vi "KE622x -- Set Current Level.vi"(0 "Resource In":refnum<visa-resource-name>, 1 "Check For SCPI Errors? (T)":bool=TRUE, 7 "Current Level (A) In":T1=0.1 min=-0.105 max=0.105 format="%.4p", 11 "error in (no error)":errorcluster, 12 "Read Back Set Value? (T)":bool=TRUE) -> (4 "Resource Out (dupl)":refnum<visa-resource-name>, 8 "Current Level (A) Out":T1=0.1 min=-0.105 max=0.105 format="%.4p", 15 "error out":errorcluster)   [LabVIEW 2019, in "Keithley 622x.lvlib"]
doc: "Sets the output current level when the source is operating in a DC mode (i.e. static mode)."
uses:
  Keithley 622x.lvlib
  Typedefs/KE622x -- Current Level.ctl
  Typedefs/KE622x -- Current Ranges.ctl
  Typedefs/KE622x -- Current Range.ctl
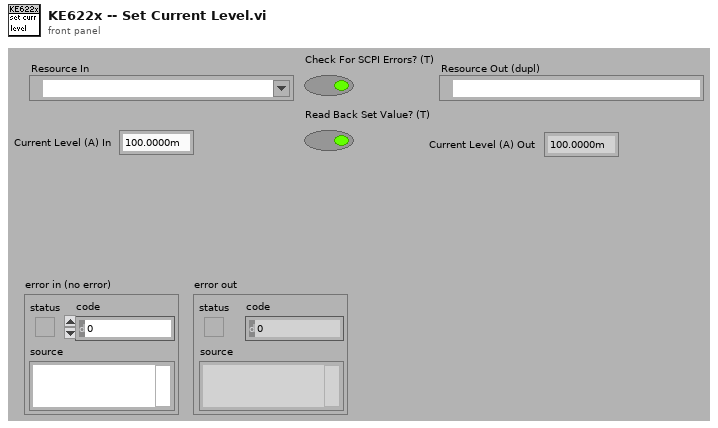
[diagram p1: front panel]
types:
  T1 = typedef "Keithley 622x.lvlib/KE622x -- Current Level.ctl" = dbl
  T2 = typedef "Keithley 622x.lvlib/KE622x -- Current Range.ctl" = cluster{"Auto Range?":bool, "Man / Selected\nRange":T3}
  T3 = typedef "Keithley 622x.lvlib/KE622x -- Current Ranges.ctl" = enum16{"2nA", "20nA", "200nA", "2uA", "20uA", "200uA", "2mA", "20mA", "100mA"}
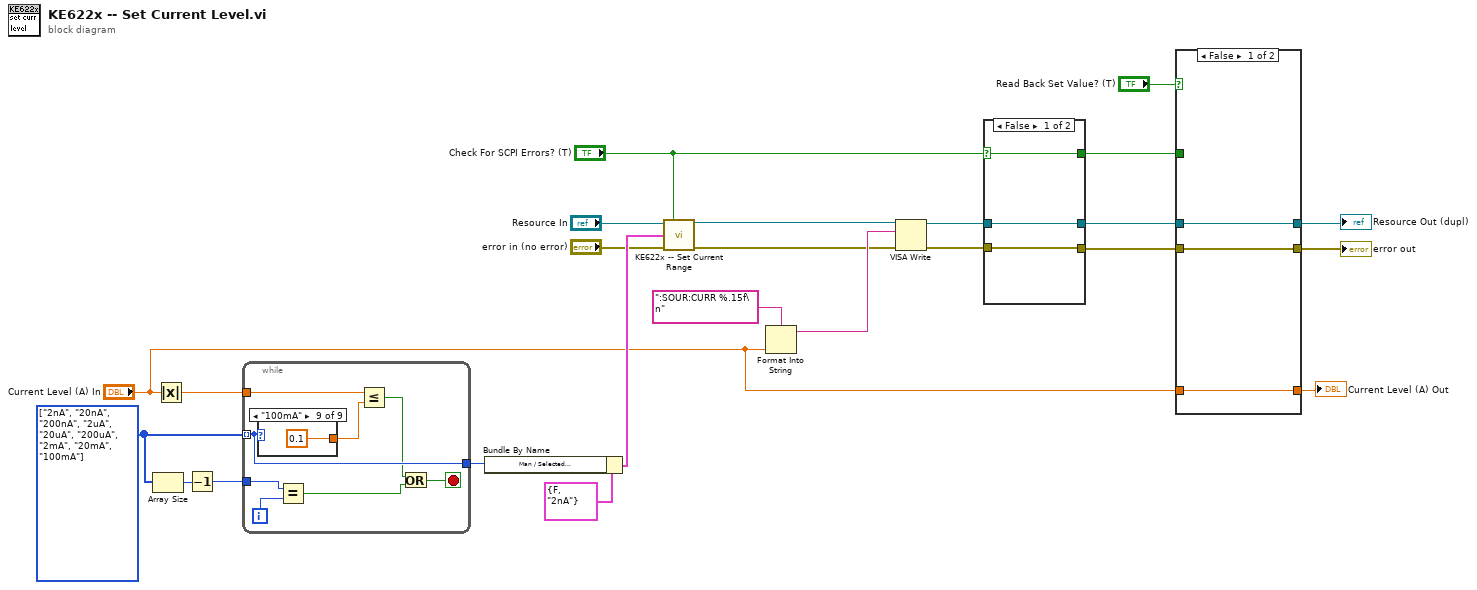
[diagram p0: block diagram]
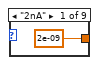
[diagram p2: hidden frame]
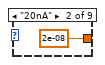
[diagram p3: hidden frame]
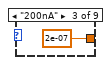
[diagram p4: hidden frame]
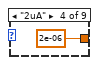
[diagram p5: hidden frame]
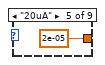
[diagram p6: hidden frame]
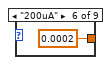
[diagram p7: hidden frame]
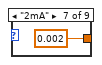
[diagram p8: hidden frame]
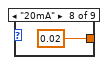
[diagram p9: hidden frame]
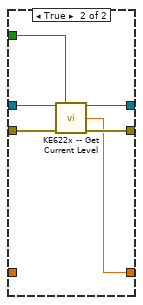
[diagram p10: hidden frame]
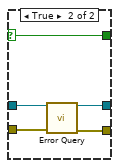
[diagram p11: hidden frame]
diagram:
  w10 = T3[] [enum."2nA", enum."20nA", enum."200nA", enum."2uA", enum."20uA", enum."200uA", enum."2mA", enum."20mA", enum."100mA"] items=["2nA", "20nA", "200nA", "2uA", "20uA", "200uA", "2mA", "20mA", "100mA"]
  n1 = Array Size(array=w10) -> (size(s)=w9:i32)
  n2 = Absolute Value(x="Current Level (A) In") -> (abs(x)=w11:T1)
  n3 = Decrement(x=w9) -> (x-1=w8:i32)
  n4 = while {
    tunnel: w11 -> [w32]
    tunnel: w10 -> [w31] mode=indexing
    tunnel: [w31] -> w6
    tunnel: w8 -> [w27]
    i -> [w28]
    stop <- w26 stop-if-true
    n5 = case shown="\"100mA\"" w31 {
      tunnel: [2e-09 2e-08 2e-07 2e-06 2e-05 0.0002 0.002 0.02 0.1] -> w30
      frame "2nA" {
      }
      frame "20nA" {
      }
      frame "200nA" {
      }
      frame "2uA" {
      }
      frame "20uA" {
      }
      frame "200uA" {
      }
      frame "2mA" {
      }
      frame "20mA" {
      }
      frame "100mA" {
      }
    }
    n6 = Equal?(x=w27, y=w28) -> (x = y?=w25:bool)
    n7 = Less Or Equal?(x=w32, y=w30) -> (x <= y?=w29:bool)
    n8 = Or(x=w29, y=w25) -> (x .or. y?=w26:bool)
  }
  n9 = Bundle By Name(cluster=T2 {"Auto Range?"=FALSE, "Man / Selected\nRange"=enum."2nA"} ("Current Range In"), "Man / Selected\nRange"=w6) -> (w5:T2)
  n10 = call "KE622x -- Set Current Range.vi"("Resource In"="Resource In", "Check For SCPI Errors? (T)"="Check For SCPI Errors? (T)", "Current Range In"=w5, "error in (no error)"="error in (no error)") -> ("Resource Out (dupl)"=w1:refnum<visa-resource-name>, "error out"=w2:errorcluster)  [unwired: 9 in, 1 out]
  n11 = Format Into String(format string=":SOUR:CURR %.15f\n", "Current Level (A) In") -> (resulting string=w23:string)  [unwired: 2 in, 1 out]
  n12 = VISA Write(VISA resource name=w1, write buffer=w23, error in (no error)=w2) -> (VISA resource name out=w22:refnum<visa-resource-name>, error out=w21:errorcluster)  [unwired: 1 out]
  n13 = case shown="False" "Check For SCPI Errors? (T)" {
    selector: "Check For SCPI Errors? (T)" -> [w42 w45]
    tunnel: w22 -> [w44 w49]
    tunnel: w21 -> [w43 w48]
    tunnel: [w43 w47] -> w17
    tunnel: [w44 w46] -> w18
    tunnel: [w42 w45] -> w16
    frame False {
    }
    frame True {
      n14 = call "Error Query.vi"("VISA Resource In"=w49, "error in (no error)"=w48) -> ("VISA Resource Out (dupl)"=w46:refnum<visa-resource-name>, "error out"=w47:errorcluster)  [unwired: 10 in, 2 out]
    }
  }
  n15 = case shown="False" "Read Back Set Value? (T)" {
    tunnel: "Current Level (A) In" -> [w50 _]
    tunnel: [w50 w53] -> w19
    tunnel: w18 -> [w52 w58]
    tunnel: w17 -> [w51 w57]
    tunnel: w16 -> [_ w56]
    tunnel: [w52 w55] -> w15
    tunnel: [w51 w54] -> w14
    frame False {
    }
    frame True {
      n16 = call "KE622x -- Get Current Level.vi"("Resource In"=w58, "Check For SCPI Errors? (T)"=w56, "error in (no error)"=w57) -> ("Resource Out (dupl)"=w55:refnum<visa-resource-name>, "Current Level (A)"=w53:T1, "error out"=w54:errorcluster)  [unwired: 10 in]
    }
  }
  "Resource Out (dupl)" <- w15
  "error out" <- w14
  "Current Level (A) Out" <- w19
